vi "Riccati_Check_Stabilizable.vi"(9 "B":T1, 11 "A":T1) -> (0 "Error":errorcluster, 3 "Bad":bool)   [LabVIEW 2019, in "Trajectory_Library.lvlib"]
uses:
  Trajectory_Library.lvlib
  <vilib>/Analysis/Matrix/Datatypes/RealMatrix.ctl
  <vilib>/Analysis/Matrix/NI_Matrix.lvlib
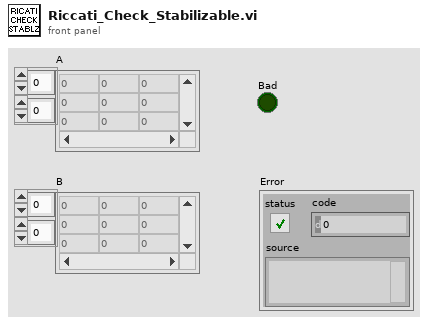
[diagram p1: front panel]
types:
  T1 = typedef "NI_Matrix.lvlib/RealMatrix.ctl" = dbl[][]
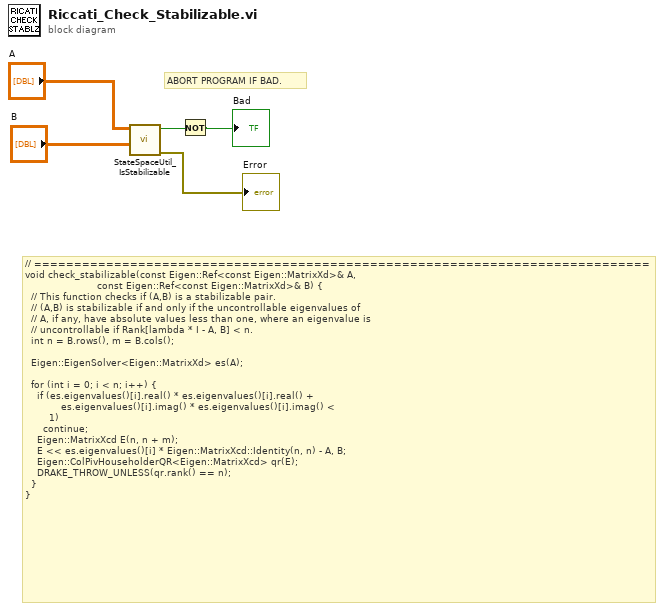
[diagram p0: block diagram]
diagram:
  # "// =============================================================================\nvoid check_stabilizable(const Eigen::Ref<const Eigen::MatrixXd>& A,\n                        const Eigen::Ref<const Eigen::MatrixXd>& B) {\n  // This function checks if (A,B) is a stabilizable pair.\n  // (A,B) is stabilizable if and only if the uncontrollable eigenvalues of\n  // A, if any, have absolute values less than one, where an eigenvalue is\n  // uncontrollable if Rank[lambda * I - A, B] < n.\n  int n = B.rows(), m = B.cols();\n\n  Eigen::EigenSolver<Eigen::MatrixXd> es(A);\n\n  for (int i = 0; i < n; i++) {\n    if (es.eigenvalues()[i].real() * es.eigenvalues()[i].real() +\n            es.eigenvalues()[i].imag() * es.eigenvalues()[i].imag() <\n        1)\n      continue;\n    Eigen::MatrixXcd E(n, n + m);\n    E << es.eigenvalues()[i] * Eigen::MatrixXcd::Identity(n, n) - A, B;\n    Eigen::ColPivHouseholderQR<Eigen::MatrixXcd> qr(E);\n    DRAKE_THROW_UNLESS(qr.rank() == n);\n  }\n}"
  # "ABORT PROGRAM IF BAD."
  n1 = call "StateSpaceUtil_IsStabilizable.vi"("B"="B", "A"="A") -> ("Error"=→"Error":errorcluster, "IsStabilizable"=w4:bool)  [unwired: 6 in, 2 out]
  n2 = Not(x=w4) -> (.not. x?=→"Bad":bool)
